vi "Build Data Validation String From String Model.vi"(10 "String Model is HEX?":bool, 11 "String Model In":string) -> (2 "Regular Expression":string, 3 "String Model Out":string)   [LabVIEW 2010]
doc: "This VI creates a case sensitive regular expression based on the String Model In input."
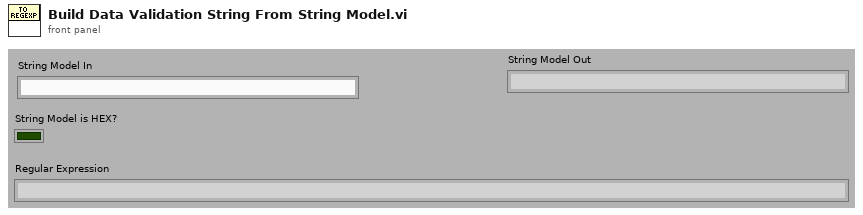
[diagram p1: front panel]
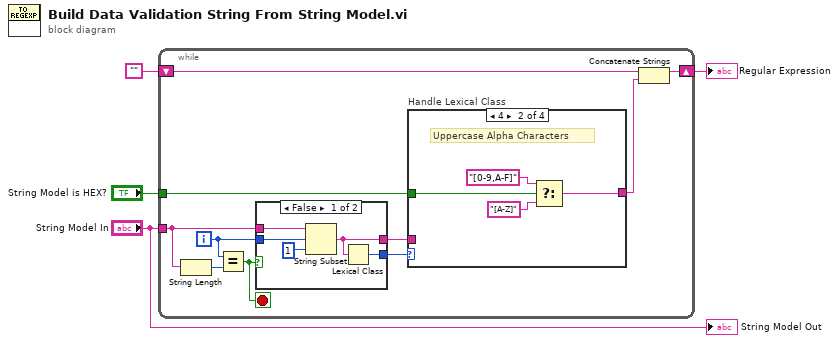
[diagram p0: block diagram]
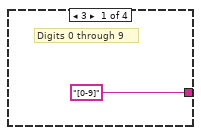
[diagram p2: hidden frame]
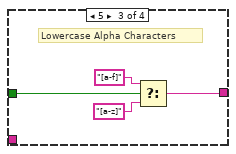
[diagram p3: hidden frame]
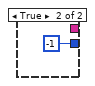
[diagram p5: hidden frame]
diagram:
  n1 = while {
    tunnel: "String Model In" -> [w14]
    shift-right: [w7] -> w3
    shift-left: "" -> [w8]
    tunnel: "String Model is HEX?" -> [w5]
    i -> [w12]
    stop <- w11 stop-if-true
    n2 = String Length(string=w14) -> (length=w13:i32)
    n3 = Equal?(x=w12, y=w13) -> (x = y?=w11:bool)
    n4 = case shown="False" w11 {
      tunnel: [w28 i16 -1] -> w10
      tunnel: w14 -> [w27 _]
      tunnel: w12 -> [w26 _]
      tunnel: [w25 _] -> w9
      frame False {
        n5 = String Subset(string=w27, offset (0)=w26, length (rest)=1 ("length (rest)")) -> (substring=w25:string)
        n6 = Lexical Class(1:w25) -> (0:w28:i16)
      }
      frame True {
      }
    }
    n7 = case "Handle Lexical Class" shown="4" w10 {
      tunnel: w9 -> [_ _ _ w24]
      tunnel: ["[0-9]" w18 w23 w24] -> w6
      tunnel: w5 -> [_ w16 w20 _]
      frame 3 {
        # "Digits 0 through 9"
      }
      frame 4 {
        # "Uppercase Alpha Characters"
        n8 = Select(t="[0-9,A-F]", s=w16, f="[A-Z]") -> (s? t:f=w18:string)
      }
      frame 5 {
        # "Lowercase Alpha Characters"
        n9 = Select(t="[a-f]", s=w20, f="[a-z]") -> (s? t:f=w23:string)
      }
      frame 6, Default {
        # "All Other characters"
      }
    }
    n10 = Concatenate Strings(w8, w6) -> (w7:string)
  }
  "Regular Expression" <- w3
  "String Model Out" <- "String Model In"
